vi "svx_Oct_Space Markers.vi"(9 "Z Scale Graph ref":refnum<vi>, 11 "markers in":dbl[](array[numeric])) -> (1 "Z Scale Graph ref out":refnum<vi>, 3 "markers out":dbl[](array[numeric]))   [LabVIEW 2017, in "SVX Octave Waterfall Graph.xctl"]
uses:
  <vilib>/addons/_XControls/Octave Waterfall Graph/SVX Octave Waterfall Graph.xctl
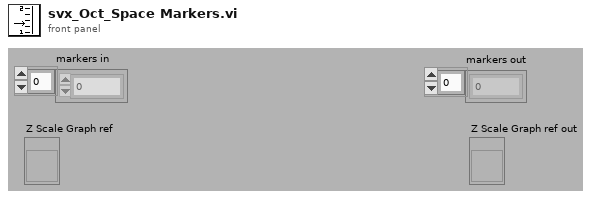
[diagram p1: front panel]
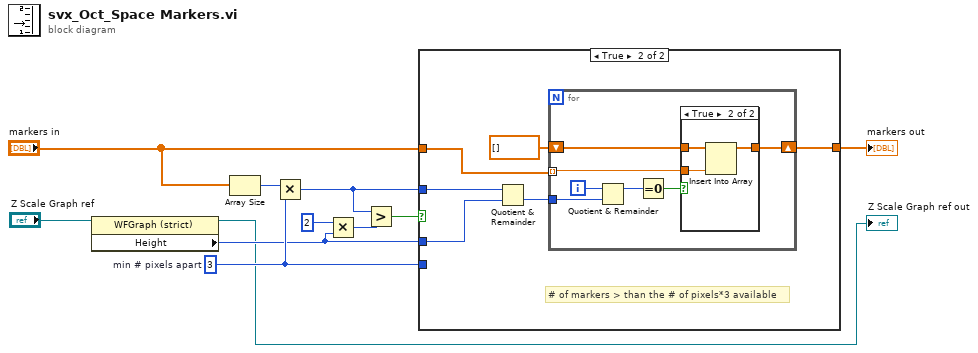
[diagram p0: block diagram]
diagram:
  w6 = u32 3  # min # pixels apart
  n1 = property on="Property Node" class="WFGraph (strict)"(reference="Z Scale Graph ref") -> (reference out=→"Z Scale Graph ref out":refnum<vi>, "Height"=w4:u32)  [unwired: 1 in, 1 out]
  n2 = Array Size(array="markers in") -> (size(s)=w7:i32)
  n3 = Multiply(x=w7, y=w6) -> (x*y=w5:u32)
  n4 = Multiply(x=u32 2 ("y"), y=w4) -> (x*y=w2:u32)
  n5 = Greater?(x=w5, y=w2) -> (0:w9:bool)
  n6 = case shown="True" w9 {
    tunnel: "markers in" -> [w12 w18]
    tunnel: [w12 w16] -> w10
    tunnel: w5 -> [_ w15]
    tunnel: w4 -> [_ w14]
    tunnel: w6 -> [_ _]
    frame False {
      # "enough spacing for the markers"
    }
    frame True {
      # "# of markers > than the # of pixels*3 available"
      n7 = Quotient & Remainder(x=w15, y=w14) -> (floor(x/y)=w13:u32)  [unwired: 1 out]
      n8 = for {
        tunnel: w18 -> [w21] mode=indexing
        shift-right: [w20] -> w16
        shift-left: dbl[] [] -> [w22]
        tunnel: w13 -> [w24]
        i -> [w25]
        n9 = Quotient & Remainder(x=w25, y=w24) -> (x-y*floor(x/y)=w23:u32)  [unwired: 1 out]
        n10 = Equal To 0?(x=w23) -> (x = 0?=w19:bool)
        n11 = case shown="True" w19 {
          tunnel: w22 -> [w26 w29]
          tunnel: w21 -> [_ w28]
          tunnel: [w26 w27] -> w20
          frame False {
          }
          frame True {
            n12 = Insert Into Array(array=w29, new element=w28) -> (w27:dbl[])  [unwired: 1 in]
          }
        }
      }
    }
  }
  "markers out" <- w10
